vi "Set Analogical to Digital Channel.vi"(8 "error in (no error)":errorcluster, 11 "CCDCamera in":refnum<class "Ixon_Ultra.lvclass">) -> (0 "error out":errorcluster, 3 "CCDCamera out":refnum<class "Ixon_Ultra.lvclass">)   [LabVIEW 2018, in "Ixon_Ultra.lvclass"]
doc: "Set Analogical to digital channel\n\nEMCCDs of the Andor have just one AD channel. So, the value of this parameter must be zero"
uses:
  Ixon_Ultra.lvclass
  C:/Users/Denis/Desktop/S4ACS/S4ACS/Simulated_CCD_Camera/Simulated Camera.lvclass
  Simulated_CCD_Camera/Simulated Camera.lvclass
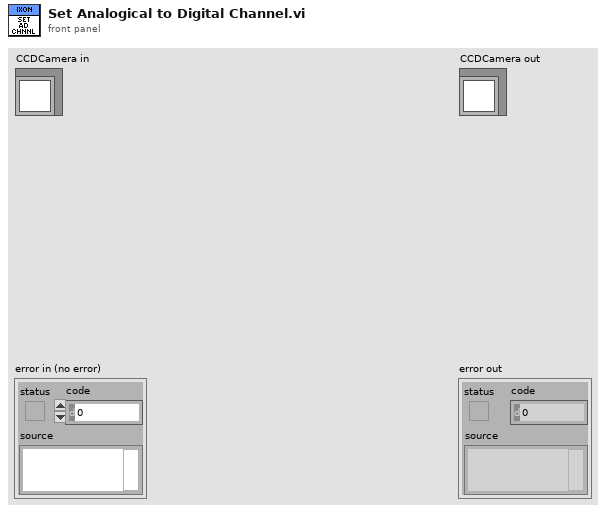
[diagram p1: front panel]
types:
  T1 = cluster{"PREAMP":u16, "READOUT_RATE":u16, "VERTICAL_SHIFT_SPEED":u16, "READ_MODE":u16, "VERTICAL_CLOCK_VOLTAGE":u16, "ACQUISITION_MODE":u16, "AD_CHANNEL":u16, "SHUTTER_TTL":u16, "SHUTTER_OPENING_TIME":u16, "SHUTTER_CLOSING_TIME":u16, "SHUTTER_MODE":u16, "TRIGGER_MODE":u16, "VBIN":u16, "INITIAL_LINE":u16, "INITIAL_COLUMN":u16, "FINAL_LINE":u16, "FINAL_COLUMN":u16, "HBIN":u16, "TEMP":i32, "COOLER_POWER_STATUS":u16}
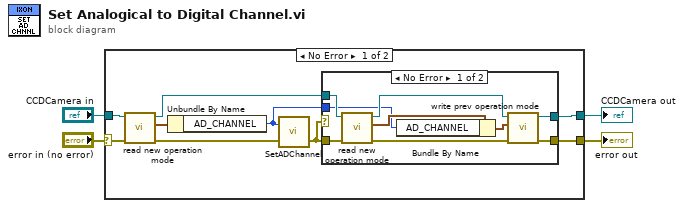
[diagram p0: block diagram]
diagram:
  n1 = case shown="No Error" "error in (no error)" {
    selector: "error in (no error)" -> [w13 w26]
    tunnel: [w9 w26] -> w4
    tunnel: [w8 w25] -> w3
    tunnel: "CCDCamera in" -> [w11 w25]
    frame No Error {
      n2 = call "read new operation mode.vi"("error in (no error)"=w13, "CCDCamera in"=w11) -> ("error out"=w5:errorcluster, "new operation mode"=w12:T1, "CCDCamera out"=w10:refnum<class "Ixon_Ultra.lvclass">)  [unwired: 7 in]
      n3 = Unbundle By Name(w12) -> ("AD_CHANNEL"=w7:u16)
      n4 = call <userlib>:"SetADChannel.vi"("error in (no error)"=w5, "channel"=w7) -> ("error out"=w6:errorcluster)  [unwired: 1 out]
      n5 = case shown="No Error" w6 {
        tunnel: [w21 w24] -> w8
        tunnel: [w19 w23] -> w9
        tunnel: w10 -> [w16 w24]
        tunnel: w6 -> [w14 w23]
        tunnel: w7 -> [w15 _]
        frame No Error {
          n6 = call "read new operation mode.vi"("error in (no error)"=w14, "CCDCamera in"=w16) -> ("error out"=w20:errorcluster, "new operation mode"=w18:T1, "CCDCamera out"=w22:refnum<class "Ixon_Ultra.lvclass">)  [unwired: 7 in]
          n7 = Bundle By Name(cluster=w18, "AD_CHANNEL"=w15) -> (w17:T1)
          n8 = call "write prev operation mode.vi"("error in (no error)"=w20, "prev operation mode"=w17, "Simulated_CCD_Camera in"=w22) -> ("error out"=w19:errorcluster, "Simulated_CCD_Camera out"=w21:refnum<class "Ixon_Ultra.lvclass">)  [unwired: 7 in]
        }
        frame Error {
        }
      }
    }
    frame Error {
    }
  }
  "error out" <- w4
  "CCDCamera out" <- w3
